vi "Load Effect Plugins.vi"() -> (3 "Effect Plugins":refnum<class "Effect Interface.lvclass">[](array[class]))   [LabVIEW 2018]
uses:
  Effect Interface/Effect Interface.lvlibp/Effect Interface Class/Effect Interface.lvclass
  <vilib>/Utility/LVLibp/NI_PackedLibraryUtility.lvlib
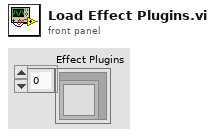
[diagram p1: front panel]
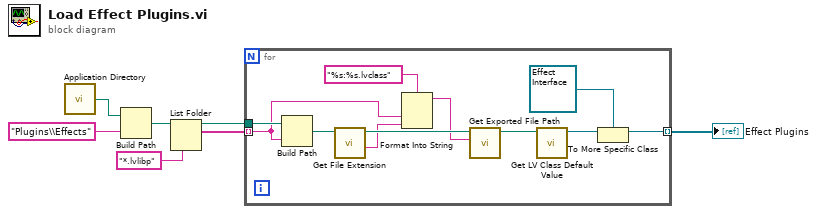
[diagram p0: block diagram]
diagram:
  n1 = call <vilib>:"Application Directory.vi"() -> ("Application Directory"=w7:path)
  n2 = Build Path(base path=w7, name or relative path="Plugins\\Effects") -> (appended path=w5:path)
  n3 = List Folder(path=w5, pattern="*.lvlibp") -> (path out=w2:path, filenames=w3:string[])  [unwired: 2 in, 2 out]
  n4 = for {
    tunnel: w3 -> [w13] mode=indexing
    tunnel: w2 -> [w18]
    tunnel: [w8] -> w1 mode=indexing
    n5 = Build Path(base path=w18, name or relative path=w13) -> (appended path=w17:path)
    n6 = call <vilib>:"Get File Extension.vi"("file"=w17) -> ("filename without extension"=w12:string, "dup file"=w16:path)  [unwired: 6 in, 3 out]
    n7 = Format Into String(format string="%s:%s.lvclass", w13, w12) -> (resulting string=w14:string)  [unwired: 2 in, 1 out]
    n8 = call <vilib>:"Get Exported File Path.vi"("qualified name"=w14, "packed library path"=w16) -> ("path"=w11:path)  [unwired: 8 in, 1 out]
    n9 = call <vilib>:"Get LV Class Default Value.vi"("class path"=w11) -> ("object"=w10:refnum<class>)  [unwired: 9 in, 1 out]
    n10 = To More Specific Class(target class=refnum<class "Effect Interface.lvclass"> refnum ("Effect Interface.lvlibp:Effect Interface.lvclass"), reference=w10) -> (specific class reference=w8:refnum<class "Effect Interface.lvclass">)  [unwired: 1 in, 1 out]
  }
  "Effect Plugins" <- w1
